vi "BRig_dataLC_Cue2_PostR_Prob_l1.vi"() -> (2 "output_Cue2_PostR_Prob":i32)   [LabVIEW 2014]
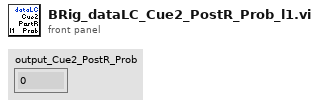
[diagram p1: front panel]
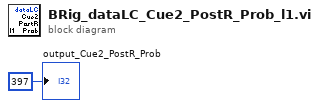
[diagram p0: block diagram]
diagram:
  "output_Cue2_PostR_Prob" <- 397 ("output_iBlock")
